vi "Build Empty ID Error.vi"(0 "Unique ID":string, 11 "Error In":errorcluster) -> (4 "Unique ID Out":string, 15 "Error Out":errorcluster)   [LabVIEW 2016, in "Tree Manager.lvclass"]
uses:
  Tree Manager.lvclass
  <vilib>/Utility/error.llb/Error Cluster From Error Code.vi
  <vilib>/ErrorRing/Error Ring.xnode
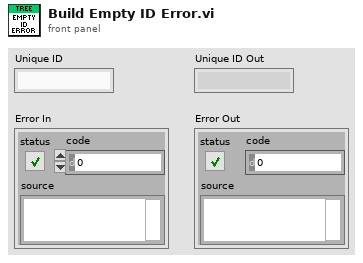
[diagram p1: front panel]
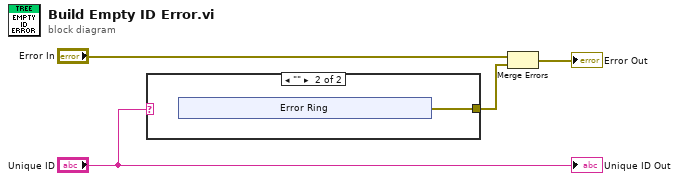
[diagram p0: block diagram]
diagram:
  n1 = case shown="\"\"" "Unique ID" {
    tunnel: [_ w5] -> w2
    frame "False", Default {
    }
    frame "" {
      n2 = xnode "Error Ring"() -> ("error out"=w5:errorcluster)
    }
  }
  n3 = Merge Errors("Error In", w2) -> (→"Error Out":errorcluster)
  "Unique ID Out" <- "Unique ID"
